vi "MB Slave Read All Input Registers (poly).vi"(5 "error in":errorcluster) -> (14 "Input Registers":u16[](array[numeric]), 19 "error out":errorcluster)   [LabVIEW 2020]
doc: "Reads all input registers from the slave's memory table."
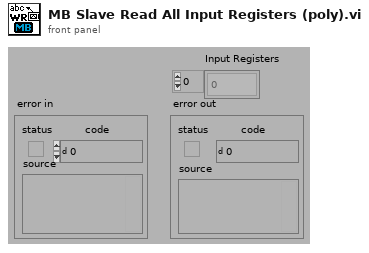
[diagram p1: front panel]
types:
  T1 = enum16{"Discrete Inputs", "Coils", "Input Registers", "Holding Registers"}
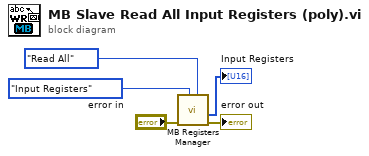
[diagram p0: block diagram]
diagram:
  n1 = call "MB Registers Manager.vi"("Function"=enum16{"Init", "Read", "Write", "Read All"}."Read All", "Table"=T1."Input Registers", "error in (no error)"="error in") -> ("error out"=→"error out":errorcluster, "Words out"=→"Input Registers":u16[])  [unwired: 4 in, 3 out]
